vi "IronPythonSave.vi"(4 "Optical Spectrum":T1, 6 "Electrical Measurement":T6, 7 "Stress Motor Position":dbl, 8 "error in (no error)":errorcluster, 9 "Instrument Configuration":T3={"Instrument"=enum."Unknown Instrument", "Configuration"="Test Configuration"}, 10 "Workspace Info":T2={"Device Name"="test", "Device Info"="test", "Path"=path "C:/Users/gio/Desktop/test Python2Workspace/python2workspace_test.pmat"}, 11 "Function":T5) -> (0 "error out":errorcluster)   [LabVIEW 2014]
uses:
  Hardware Control/Parameter Analyzer/Electrical Data.ctl
  SaveData Function.ctl
  SaveData Instrument Configuration.ctl
  Instrument Sequence/Instrument List.ctl
  SaveData Workspace Info.ctl
  Hardware Control/Spectrometer/Spectral Data.ctl
  C:/IBM OEDUS/Measurements/Save Data/IronPythonSave/IronPythonSave.dll
  IronPythonSave/IronPythonSave.dll
panel:
  out "Activity Log":string
  out "concatenated string":string
  # "LICENSED MATERIALS – PROPERTY OF IBM\nCopyright IBM Corp. 2016,\nALL RIGHTS RESERVED"
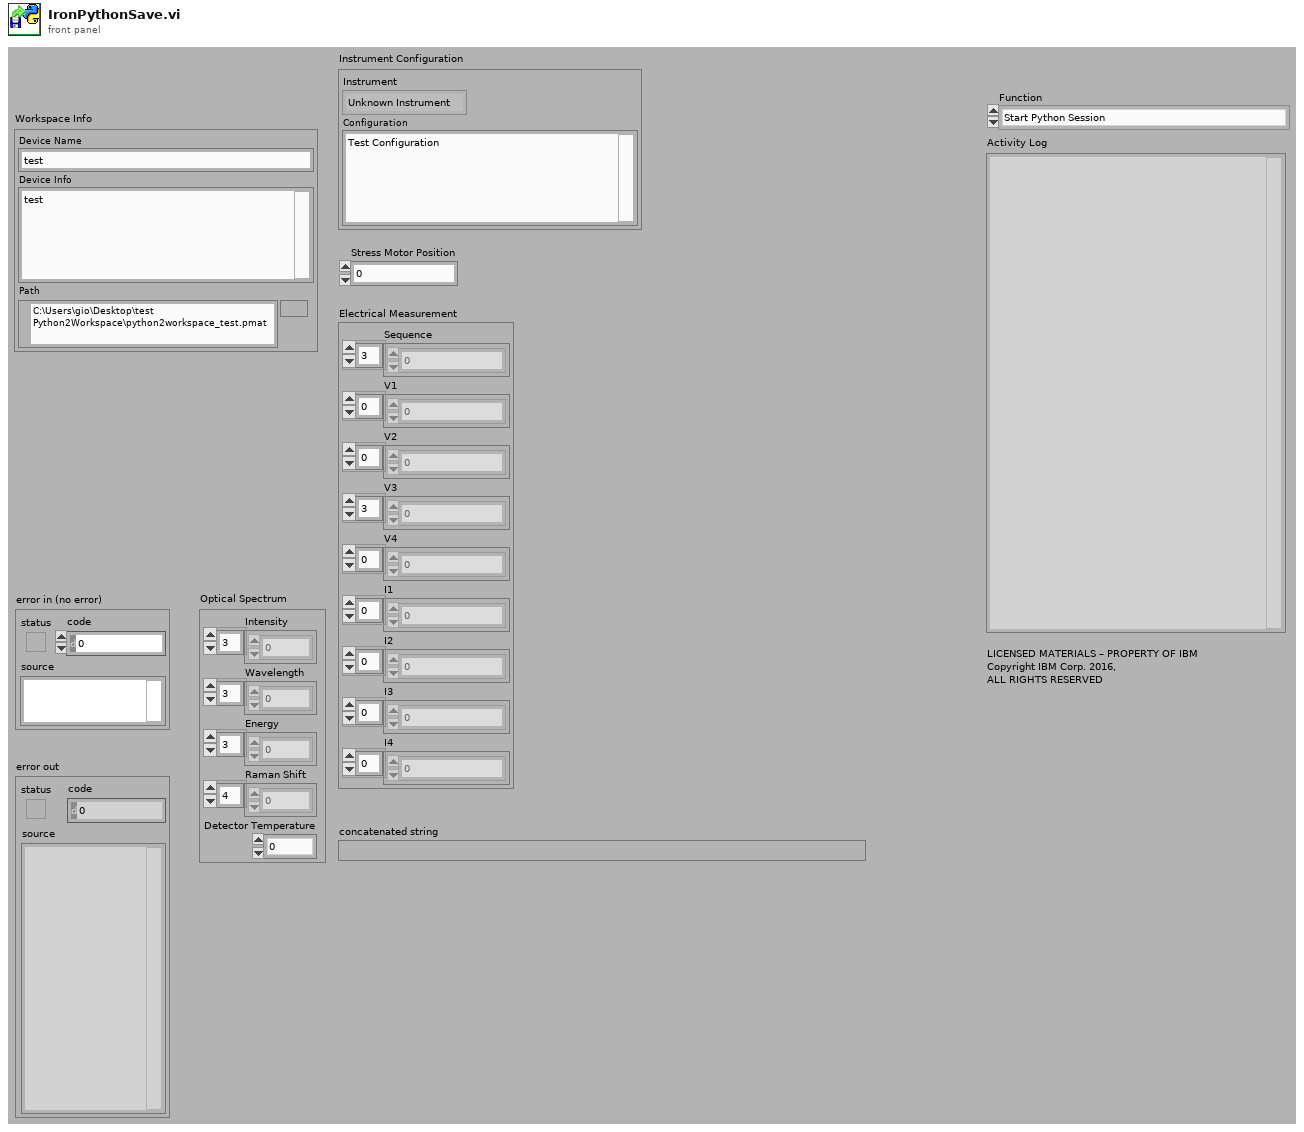
[diagram p1: front panel]
types:
  T1 = typedef "Spectral Data.ctl" = cluster{"Intensity":dbl[], "Wavelength":dbl[], "Energy":dbl[], "Raman Shift":dbl[], "Detector Temperature":dbl}
  T2 = typedef "SaveData Workspace Info.ctl" = cluster{"Device Name":string, "Device Info":string, "Path":path}
  T3 = typedef "SaveData Instrument Configuration.ctl" = cluster{"Instrument":T4, "Configuration":string}
  T4 = typedef "Instrument List.ctl" = enum32{"Unknown Instrument", "Switching Matrix", "Parameter Analyzer", "Optical Spectrometer", "Optoelectronic", "Autofocus"}
  T5 = typedef "SaveData Function.ctl" = enum16{"Start Python Session", "Set Data Structures to Default", "Append Stress Data", "Append Electrical Measurement", "Append Optical Spectrum", "Append Stress Measurement Step", "Append Instrument Sequence Step", "Set Instrument Configuration", "Set Stress Data", "Set Electrical Measurement", "Set Optical Spectum", "Save Electrical Measurement", "Save Optical Spectrum", "Save Optoelectronic Measurement", "Save Instrument Sequence", "Save Stress Measurement", "Pickle2Workspace", "Explore Variable Space", "Close"}
  T6 = typedef "Electrical Data.ctl" = cluster{"Sequence":dbl[], "V1":dbl[], "V2":dbl[], "V3":dbl[], "V4":dbl[], "I1":dbl[], "I2":dbl[], "I3":dbl[], "I4":dbl[]}
  T7 = enum32{"invalid app kind", "Development System", "Run Time System", "Student Edition", "Embedded LabVIEW", "Evaluation", "Custom"}
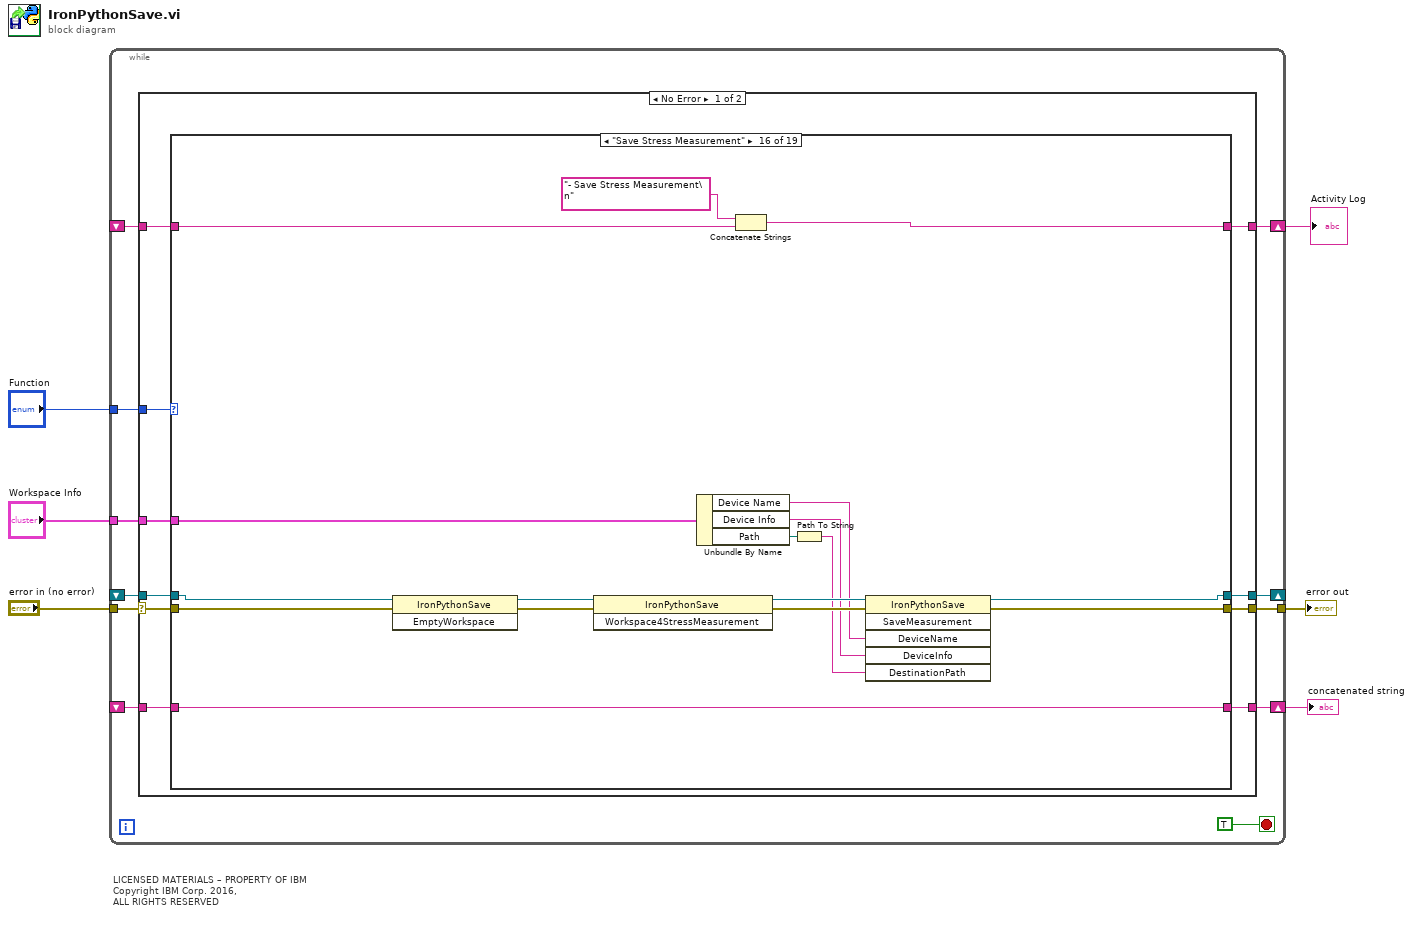
[diagram p0: block diagram]
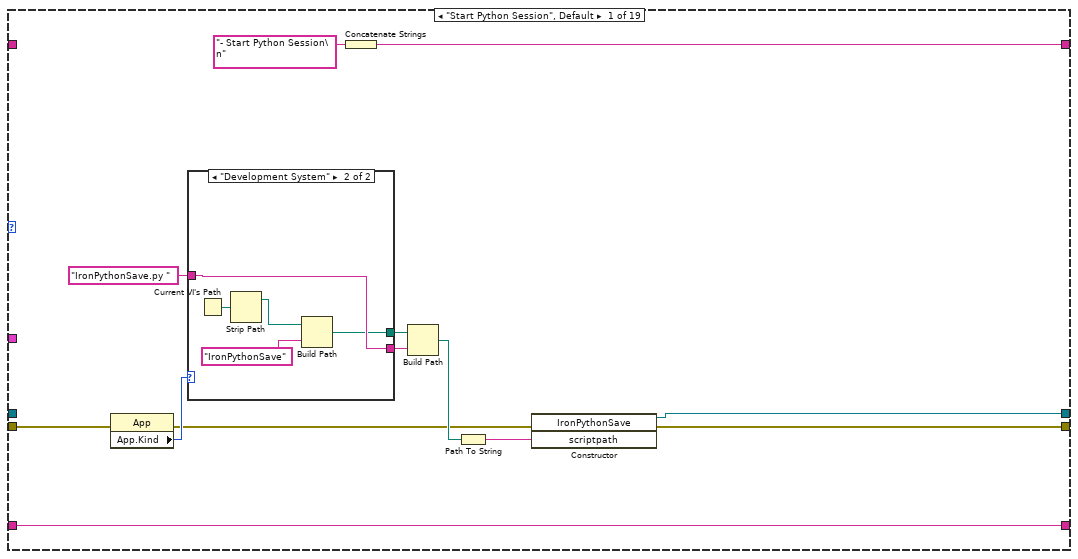
[diagram p2: hidden frame]
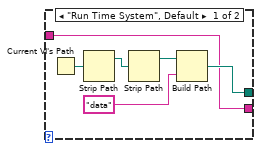
[diagram p3: hidden frame]
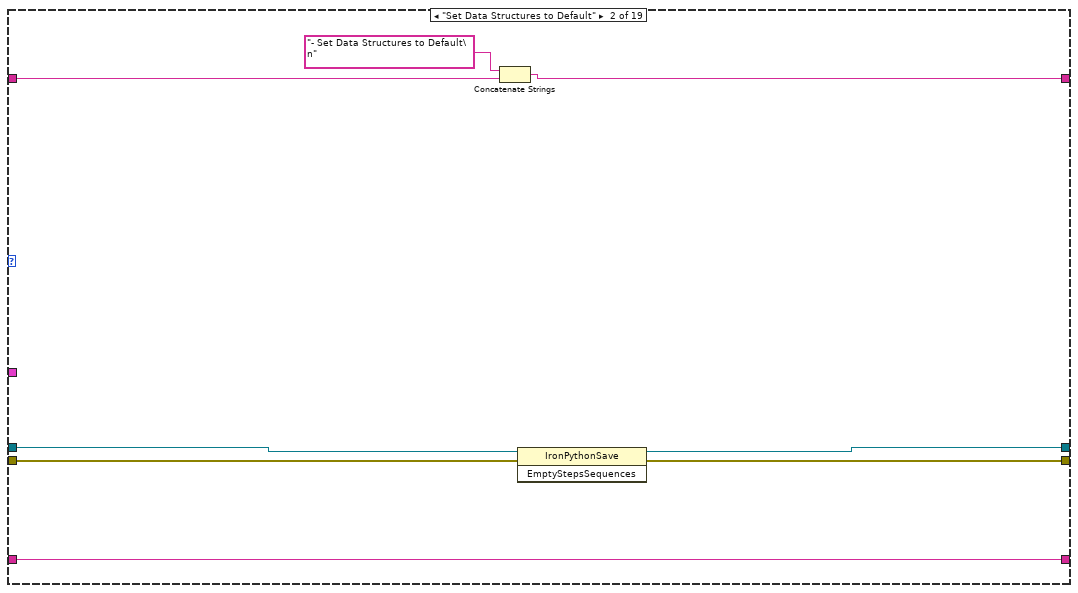
[diagram p4: hidden frame]
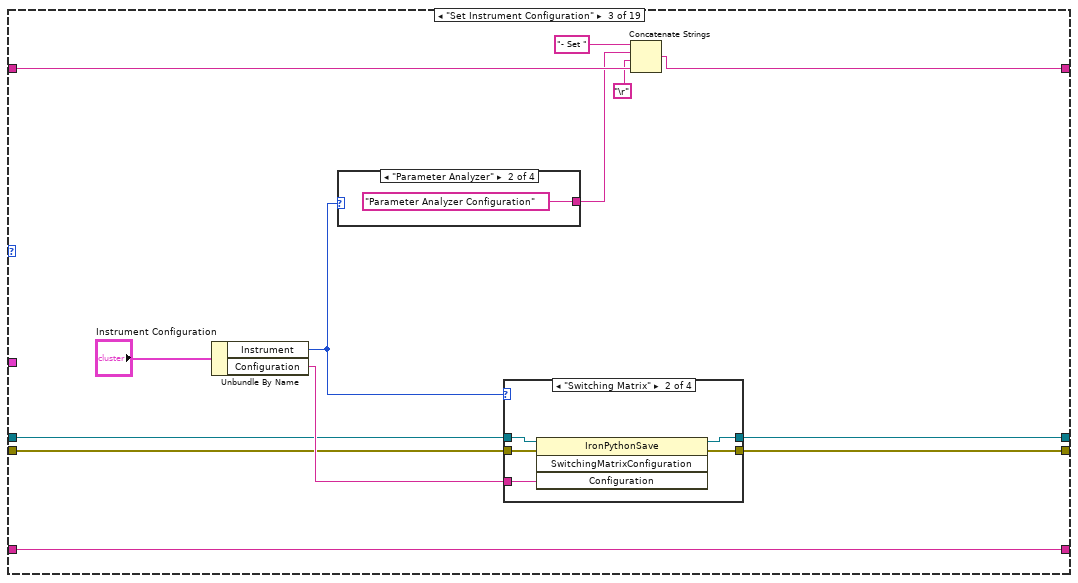
[diagram p5: hidden frame]
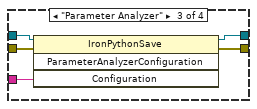
[diagram p7: hidden frame]
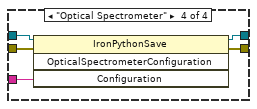
[diagram p8: hidden frame]
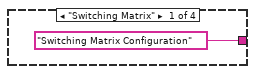
[diagram p9: hidden frame]
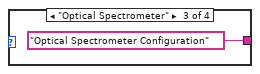
[diagram p10: hidden frame]
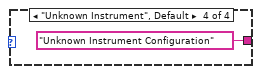
[diagram p11: hidden frame]
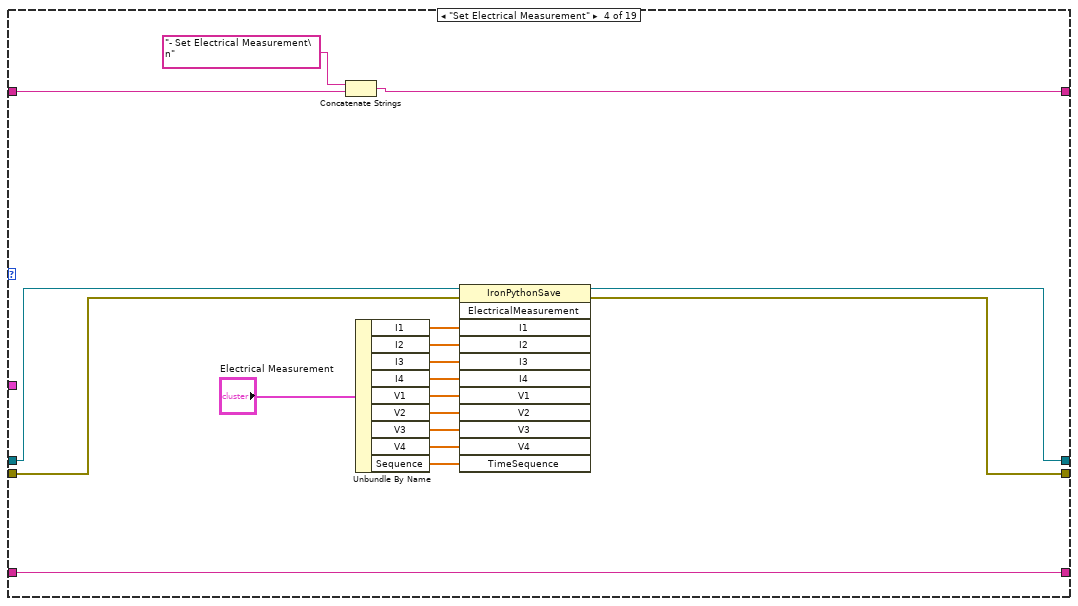
[diagram p12: hidden frame]
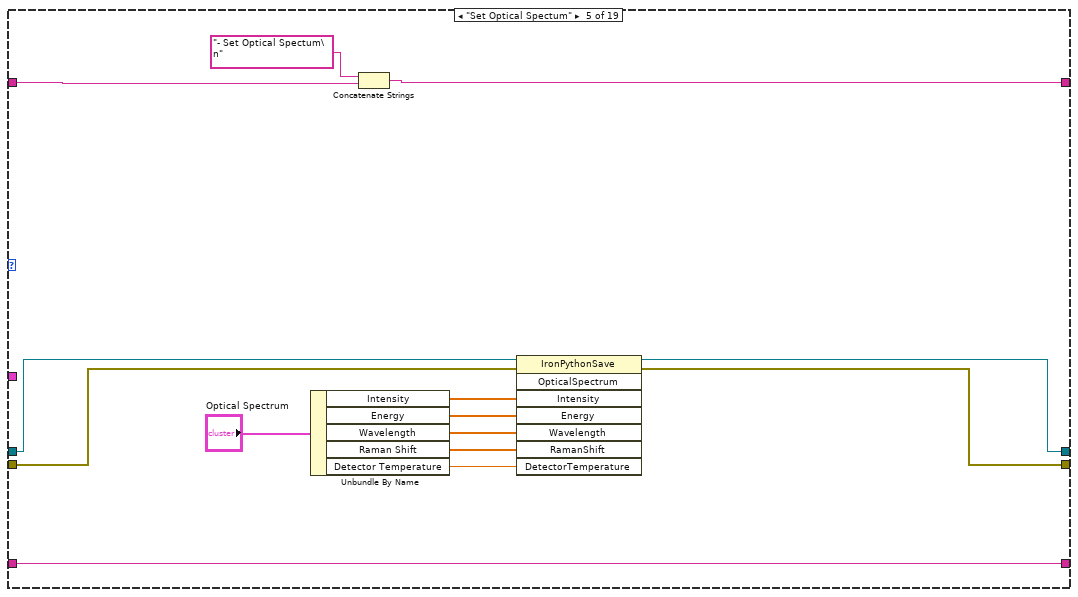
[diagram p13: hidden frame]
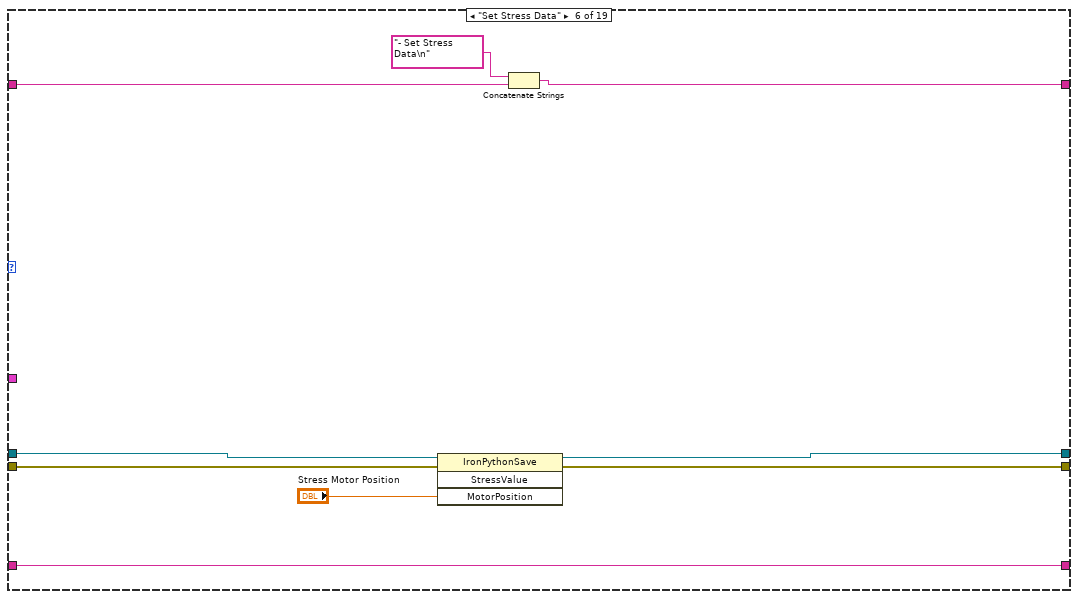
[diagram p14: hidden frame]
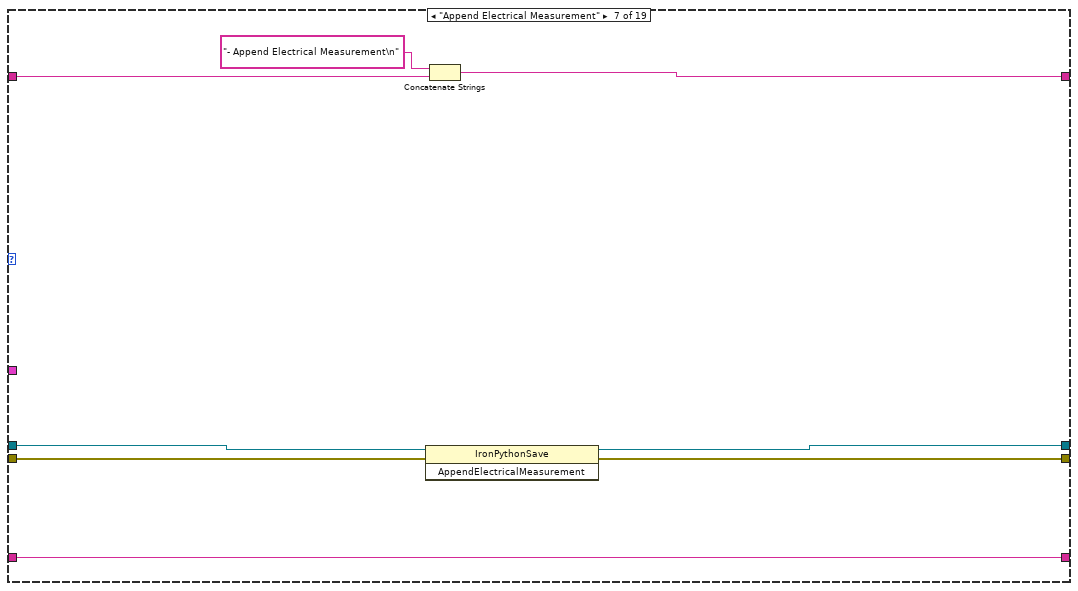
[diagram p15: hidden frame]
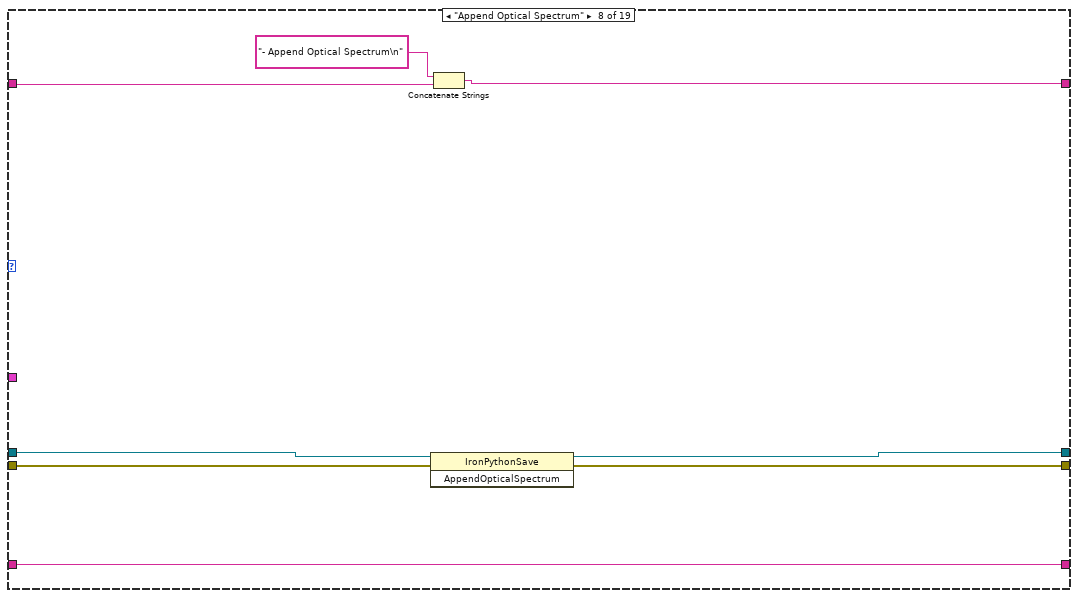
[diagram p16: hidden frame]
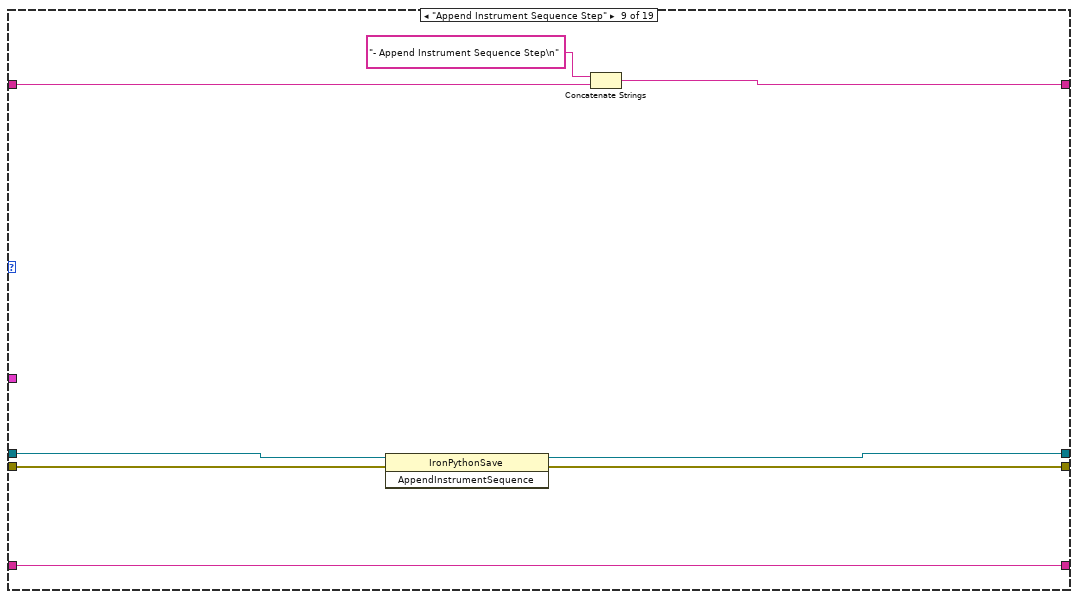
[diagram p17: hidden frame]
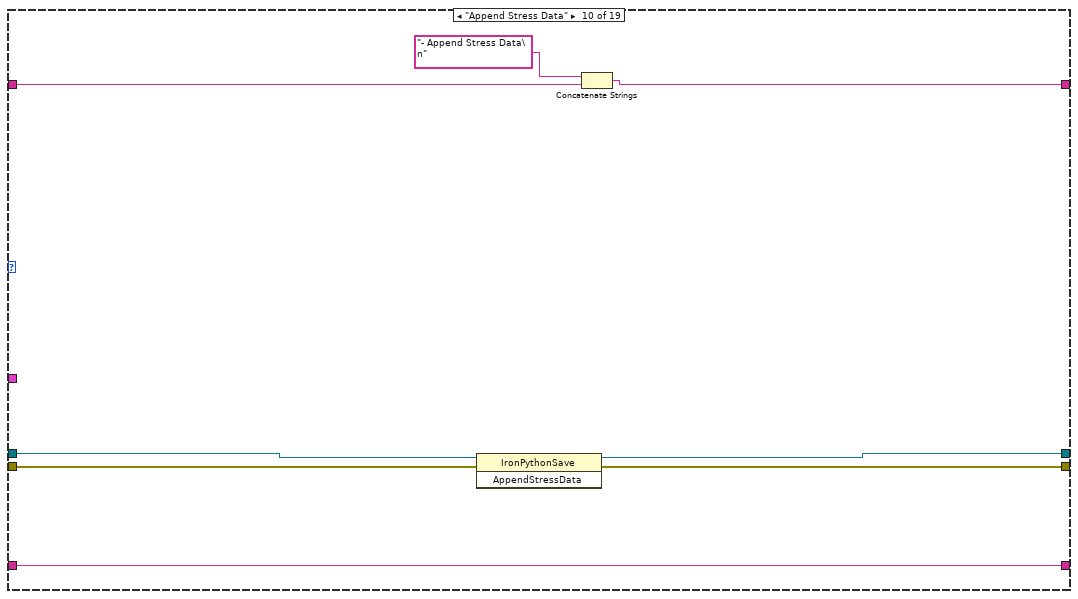
[diagram p18: hidden frame]
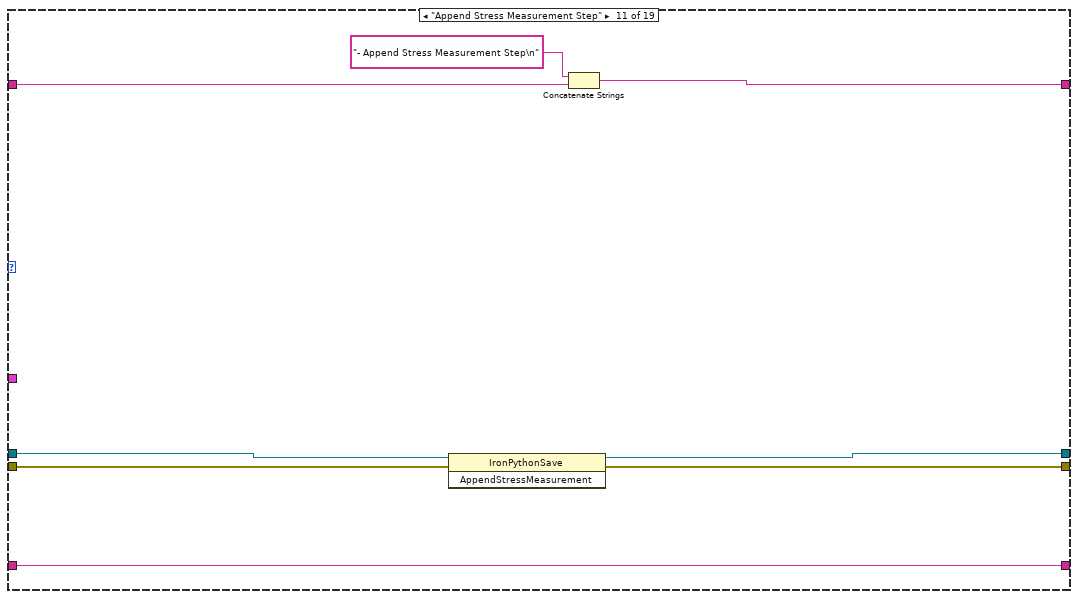
[diagram p19: hidden frame]
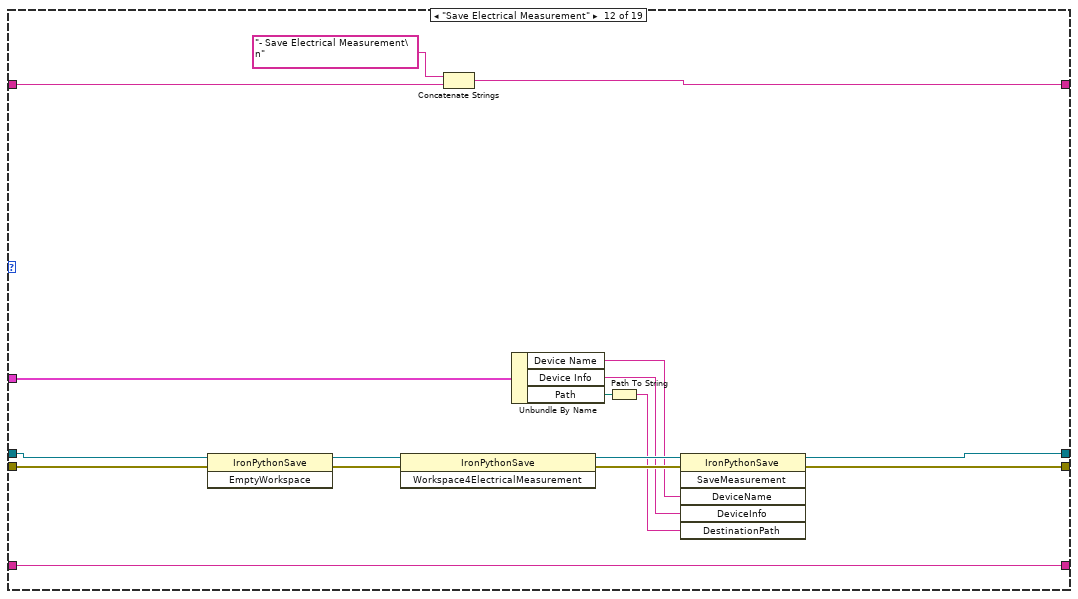
[diagram p20: hidden frame]
diagram:
  # "LICENSED MATERIALS – PROPERTY OF IBM\nCopyright IBM Corp. 2016,\nALL RIGHTS RESERVED"
  n1 = while {
    tunnel: "Workspace Info" -> [w17]
    tunnel: "Function" -> [w16]
    tunnel: [w15] -> w5
    tunnel: "error in (no error)" -> [w7]
    shift-right: [w13] -> _
    shift-left: _ -> [w12]
    shift-right: [w11] -> w2
    shift-left: _ -> [w10]
    shift-right: [w9] -> w1
    shift-left: _ -> [w8]
    stop <- TRUE stop-if-true
    n2 = case shown="No Error" w7 {
      selector: w7 -> [w24 w325]
      tunnel: w17 -> [w27 _]
      tunnel: w16 -> [w26 _]
      tunnel: [w25 w325] -> w15
      tunnel: [w23 w324] -> w13
      tunnel: w12 -> [w22 w324]
      tunnel: [w21 w323] -> w11
      tunnel: w10 -> [w20 w323]
      tunnel: w8 -> [w19 w322]
      tunnel: [w18 w322] -> w9
      frame No Error {
        n3 = case shown="\"Save Stress Measurement\"" w26 {
          tunnel: w27 -> [_ _ _ _ _ _ _ _ _ _ _ w190 w196 w217 w232 w247 _ _ w290]
          tunnel: w24 -> [w34 w54 w61 w105 w119 w129 w137 w145 w154 w161 w169 w184 w194 w216 w230 w249 w264 w269 w283]
          tunnel: [w28 w52 w64 w103 w117 w127 w136 w144 w151 w160 w167 w179 w192 w213 w229 w246 w263 w269 w288] -> w25
          tunnel: [w29 w53 w60 w104 w118 w126 w135 w143 w152 w159 w168 w178 w193 w214 w228 w245 w262 w270 w287] -> w23
          tunnel: w22 -> [_ w55 w62 w106 w120 w130 w138 w146 w153 w162 w170 w185 w195 w215 w231 w248 w262 w270 w287]
          tunnel: [w40 w59 w71 w110 w125 w134 w142 w150 w158 w166 w174 w189 w208 w227 w244 w261 w268 w272 w286] -> w21
          tunnel: w20 -> [w40 w59 w71 w110 w125 w134 w142 w150 w158 w166 w174 w189 w208 w227 w244 w261 w268 w272 _]
          tunnel: w19 -> [_ w58 w70 w109 w124 w132 w140 w148 w156 w165 w173 w188 w207 w226 w243 w260 w267 w271 w274]
          tunnel: [w39 w57 w69 w108 w123 w133 w141 w149 w157 w164 w172 w187 w206 w225 w242 w259 w266 w271 w275] -> w18
          frame "Start Python Session", Default {
            n4 = property class="App"(error in=w34) -> (error out=w31:errorcluster, "App.Kind"=w32:T7)  [unwired: 1 in, 1 out]
            n5 = case shown="\"Development System\"" w32 {
              tunnel: [w41 w50] -> w37
              tunnel: "IronPythonSave.py " ("command line") -> [w41 w50]
              tunnel: [w42 w48] -> w36
              frame "Run Time System", Default {
                n6 = Current VI's Path() -> (path=w46:path)
                n7 = Strip Path(path=w46) -> (stripped path=w45:path)  [unwired: 1 out]
                n8 = Strip Path(path=w45) -> (stripped path=w44:path)  [unwired: 1 out]
                n9 = Build Path(base path=w44, name or relative path="data" ("string")) -> (appended path=w42:path)
              }
              frame "Development System" {
                n10 = Current VI's Path() -> (path=w51:path)
                n11 = Strip Path(path=w51) -> (stripped path=w49:path)  [unwired: 1 out]
                n12 = Build Path(base path=w49, name or relative path="IronPythonSave") -> (appended path=w48:path)
              }
            }
            n13 = Concatenate Strings("- Start Python Session\n" ("string")) -> (w39:string)
            n14 = Build Path(base path=w36, name or relative path=w37) -> (appended path=w33:path)
            n15 = Path To String(path=w33) -> (string=w30:string)
            n16 = constructor class="IronPythonSave"(error in=w31, "scriptpath"=w30) -> (reference out=w29:refnum<k24>, error out=w28:errorcluster)  [unwired: 2 in, 2 out]
          }
          frame "Set Data Structures to Default" {
            n17 = Concatenate Strings("- Set Data Structures to Default\n" ("string"), w58) -> (w57:string)
            n18 = invoke class="IronPythonSave" method="EmptyStepsSequences"(reference=w55, error in=w54) -> (reference out=w53:refnum<k24>, error out=w52:errorcluster)  [unwired: 1 in, 1 out]
          }
          frame "Set Instrument Configuration" {
            n19 = Unbundle By Name("Instrument Configuration") -> ("Instrument"=w63:T4, "Configuration"=w65:string)
            n20 = case shown="\"Parameter Analyzer\"" w63 {
              tunnel: ["Switching Matrix Configuration" ("variable name") "Parameter Analyzer Configuration" ("variable name") "Optical Spectrometer Configuration" ("variable name") "Unknown Instrument Configuration" ("variable name")] -> w66
              frame "Switching Matrix" {
              }
              frame "Parameter Analyzer" {
              }
              frame "Optical Spectrometer" {
              }
              frame "Unknown Instrument", Default {
              }
            }
            n21 = case shown="\"Switching Matrix\"" w63 {
              tunnel: [w74 w76 w80 w86] -> w64
              tunnel: w65 -> [_ w75 w84 w85]
              tunnel: w62 -> [w73 w79 w82 w89]
              tunnel: w61 -> [w74 w78 w83 w88]
              tunnel: [w73 w77 w81 w87] -> w60
              frame "Unknown Instrument", Default {
              }
              frame "Switching Matrix" {
                n22 = invoke class="IronPythonSave" method="SwitchingMatrixConfiguration"(reference=w79, error in=w78, "Configuration"=w75) -> (reference out=w77:refnum<k24>, error out=w76:errorcluster)  [unwired: 1 in, 2 out]
              }
              frame "Parameter Analyzer" {
                n23 = invoke class="IronPythonSave" method="ParameterAnalyzerConfiguration"(reference=w82, error in=w83, "Configuration"=w84) -> (reference out=w81:refnum<k24>, error out=w80:errorcluster)  [unwired: 1 in, 2 out]
              }
              frame "Optical Spectrometer" {
                n24 = invoke class="IronPythonSave" method="OpticalSpectrometerConfiguration"(reference=w89, error in=w88, "Configuration"=w85) -> (reference out=w87:refnum<k24>, error out=w86:errorcluster)  [unwired: 1 in, 2 out]
              }
            }
            n25 = Concatenate Strings("- Set " ("string"), w66, "\r", w70) -> (w69:string)
          }
          frame "Set Electrical Measurement" {
            n26 = Concatenate Strings("- Set Electrical Measurement\n" ("string"), w109) -> (w108:string)
            n27 = Unbundle By Name("Electrical Measurement") -> ("I1"=w102:dbl[], "I2"=w101:dbl[], "I3"=w100:dbl[], "I4"=w99:dbl[], "V1"=w98:dbl[], "V2"=w97:dbl[], "V3"=w96:dbl[], "V4"=w95:dbl[], "Sequence"=w94:dbl[])
            n28 = invoke class="IronPythonSave" method="ElectricalMeasurement"(reference=w106, error in=w105, "I1"=w102, "I2"=w101, "I3"=w100, "I4"=w99, "V1"=w98, "V2"=w97, "V3"=w96, "V4"=w95, "TimeSequence"=w94) -> (reference out=w104:refnum<k24>, error out=w103:errorcluster)  [unwired: 1 in, 10 out]
          }
          frame "Set Optical Spectum" {
            n29 = Unbundle By Name("Optical Spectrum") -> ("Intensity"=w116:dbl[], "Energy"=w115:dbl[], "Wavelength"=w114:dbl[], "Raman Shift"=w113:dbl[], "Detector Temperature"=w112:dbl)
            n30 = Concatenate Strings("- Set Optical Spectum\n" ("string"), w124) -> (w123:string)
            n31 = invoke class="IronPythonSave" method="OpticalSpectrum"(reference=w120, error in=w119, "Intensity"=w116, "Energy"=w115, "Wavelength"=w114, "RamanShift"=w113, "DetectorTemperature"=w112) -> (reference out=w118:refnum<k24>, error out=w117:errorcluster)  [unwired: 1 in, 6 out]
          }
          frame "Set Stress Data" {
            n32 = invoke class="IronPythonSave" method="StressValue"(reference=w130, error in=w129, "MotorPosition"="Stress Motor Position") -> (reference out=w126:refnum<k24>, error out=w127:errorcluster)  [unwired: 1 in, 2 out]
            n33 = Concatenate Strings("- Set Stress Data\n" ("string"), w132) -> (w133:string)
          }
          frame "Append Electrical Measurement" {
            n34 = invoke class="IronPythonSave" method="AppendElectricalMeasurement"(reference=w138, error in=w137) -> (reference out=w135:refnum<k24>, error out=w136:errorcluster)  [unwired: 1 in, 1 out]
            n35 = Concatenate Strings("- Append Electrical Measurement\n" ("string"), w140) -> (w141:string)
          }
          frame "Append Optical Spectrum" {
            n36 = invoke class="IronPythonSave" method="AppendOpticalSpectrum"(reference=w146, error in=w145) -> (reference out=w143:refnum<k24>, error out=w144:errorcluster)  [unwired: 1 in, 1 out]
            n37 = Concatenate Strings("- Append Optical Spectrum\n" ("string"), w148) -> (w149:string)
          }
          frame "Append Instrument Sequence Step" {
            n38 = invoke class="IronPythonSave" method="AppendInstrumentSequence"(reference=w153, error in=w154) -> (reference out=w152:refnum<k24>, error out=w151:errorcluster)  [unwired: 1 in, 1 out]
            n39 = Concatenate Strings("- Append Instrument Sequence Step\n" ("string"), w156) -> (w157:string)
          }
          frame "Append Stress Data" {
            n40 = invoke class="IronPythonSave" method="AppendStressData"(reference=w162, error in=w161) -> (reference out=w159:refnum<k24>, error out=w160:errorcluster)  [unwired: 1 in, 1 out]
            n41 = Concatenate Strings("- Append Stress Data\n" ("string"), w165) -> (w164:string)
          }
          frame "Append Stress Measurement Step" {
            n42 = invoke class="IronPythonSave" method="AppendStressMeasurement"(reference=w170, error in=w169) -> (reference out=w168:refnum<k24>, error out=w167:errorcluster)  [unwired: 1 in, 1 out]
            n43 = Concatenate Strings("- Append Stress Measurement Step\n" ("string"), w173) -> (w172:string)
          }
          frame "Save Electrical Measurement" {
            n44 = invoke class="IronPythonSave" method="EmptyWorkspace"(reference=w185, error in=w184) -> (reference out=w183:refnum<k24>, error out=w182:errorcluster)  [unwired: 1 in, 1 out]
            n45 = invoke class="IronPythonSave" method="Workspace4ElectricalMeasurement"(reference=w183, error in=w182) -> (reference out=w181:refnum<k24>, error out=w180:errorcluster)  [unwired: 1 in, 1 out]
            n46 = Concatenate Strings("- Save Electrical Measurement\n" ("string"), w188) -> (w187:string)
            n47 = Unbundle By Name(w190) -> ("Device Name"=w177:string, "Device Info"=w176:string, "Path"=w191:path)
            n48 = Path To String(path=w191) -> (string=w175:string)
            n49 = invoke class="IronPythonSave" method="SaveMeasurement"(reference=w181, error in=w180, "DeviceName"=w177, "DeviceInfo"=w176, "DestinationPath"=w175) -> (reference out=w178:refnum<k24>, error out=w179:errorcluster)  [unwired: 1 in, 4 out]
          }
          frame "Save Optical Spectrum" {
            n50 = invoke class="IronPythonSave" method="EmptyWorkspace"(reference=w195, error in=w194) -> (reference out=w203:refnum<k24>, error out=w202:errorcluster)  [unwired: 1 in, 1 out]
            n51 = invoke class="IronPythonSave" method="Workspace4OpticalSPectrum"(reference=w203, error in=w202) -> (reference out=w201:refnum<k24>, error out=w200:errorcluster)  [unwired: 1 in, 1 out]
            n52 = Concatenate Strings("- Save Optical Spectrum\n" ("string"), w207) -> (w206:string)
            n53 = Unbundle By Name(w196) -> ("Device Name"=w199:string, "Device Info"=w198:string, "Path"=w204:path)
            n54 = Path To String(path=w204) -> (string=w197:string)
            n55 = invoke class="IronPythonSave" method="SaveMeasurement"(reference=w201, error in=w200, "DeviceName"=w199, "DeviceInfo"=w198, "DestinationPath"=w197) -> (reference out=w193:refnum<k24>, error out=w192:errorcluster)  [unwired: 1 in, 4 out]
          }
          frame "Save Optoelectronic Measurement" {
            n56 = invoke class="IronPythonSave" method="EmptyWorkspace"(reference=w215, error in=w216) -> (reference out=w209:refnum<k24>, error out=w210:errorcluster)  [unwired: 1 in, 1 out]
            n57 = invoke class="IronPythonSave" method="Workspace4ElectricalMeasurement"(reference=w209, error in=w210) -> (reference out=w212:refnum<k24>, error out=w211:errorcluster)  [unwired: 1 in, 1 out]
            n58 = Concatenate Strings("- Save Optoelectronic Measurement\n" ("string"), w226) -> (w225:string)
            n59 = invoke class="IronPythonSave" method="Workspace4OpticalSPectrum"(reference=w212, error in=w211) -> (reference out=w222:refnum<k24>, error out=w221:errorcluster)  [unwired: 1 in, 1 out]
            n60 = Unbundle By Name(w217) -> ("Device Name"=w220:string, "Device Info"=w219:string, "Path"=w223:path)
            n61 = Path To String(path=w223) -> (string=w218:string)
            n62 = invoke class="IronPythonSave" method="SaveMeasurement"(reference=w222, error in=w221, "DeviceName"=w220, "DeviceInfo"=w219, "DestinationPath"=w218) -> (reference out=w214:refnum<k24>, error out=w213:errorcluster)  [unwired: 1 in, 4 out]
          }
          frame "Save Instrument Sequence" {
            n63 = invoke class="IronPythonSave" method="EmptyWorkspace"(reference=w231, error in=w230) -> (reference out=w239:refnum<k24>, error out=w238:errorcluster)  [unwired: 1 in, 1 out]
            n64 = invoke class="IronPythonSave" method="Workspace4InstrumentSequence"(reference=w239, error in=w238) -> (reference out=w237:refnum<k24>, error out=w236:errorcluster)  [unwired: 1 in, 1 out]
            n65 = Unbundle By Name(w232) -> ("Device Name"=w235:string, "Device Info"=w234:string, "Path"=w240:path)
            n66 = Concatenate Strings("- Save Instrument Sequence\n" ("string"), w243) -> (w242:string)
            n67 = Path To String(path=w240) -> (string=w233:string)
            n68 = invoke class="IronPythonSave" method="SaveMeasurement"(reference=w237, error in=w236, "DeviceName"=w235, "DeviceInfo"=w234, "DestinationPath"=w233) -> (reference out=w228:refnum<k24>, error out=w229:errorcluster)  [unwired: 1 in, 4 out]
          }
          frame "Save Stress Measurement" {
            n69 = invoke class="IronPythonSave" method="EmptyWorkspace"(reference=w248, error in=w249) -> (reference out=w256:refnum<k24>, error out=w255:errorcluster)  [unwired: 1 in, 1 out]
            n70 = invoke class="IronPythonSave" method="Workspace4StressMeasurement"(reference=w256, error in=w255) -> (reference out=w254:refnum<k24>, error out=w253:errorcluster)  [unwired: 1 in, 1 out]
            n71 = Unbundle By Name(w247) -> ("Device Name"=w252:string, "Device Info"=w251:string, "Path"=w257:path)
            n72 = Concatenate Strings("- Save Stress Measurement\n" ("string"), w260) -> (w259:string)
            n73 = Path To String(path=w257) -> (string=w250:string)
            n74 = invoke class="IronPythonSave" method="SaveMeasurement"(reference=w254, error in=w253, "DeviceName"=w252, "DeviceInfo"=w251, "DestinationPath"=w250) -> (reference out=w245:refnum<k24>, error out=w246:errorcluster)  [unwired: 1 in, 4 out]
          }
          frame "Close" {
            n75 = Close Reference(reference=w262, error in (no error)=w264) -> (error out=w263:errorcluster)
            n76 = Concatenate Strings("- Python session Closed\n" ("string"), w267) -> (w266:string)
          }
          frame "Explore Variable Space" {
          }
          frame "Pickle2Workspace" {
            n77 = Unbundle By Name(w290) -> ("Path"=w289:path)
            n78 = property class="App"(error in=w283) -> (error out=w277:errorcluster, "App.Kind"=w278:T7)  [unwired: 1 in, 1 out]
            n79 = Path To String(path=w289) -> (string=w280:string)
            n80 = case shown="\"Development System\"" w278 {
              tunnel: [w300 w305] -> w286
              tunnel: [w298 w303] -> w285
              tunnel: w280 -> [w297 w304]
              tunnel: [w292 w302] -> w279
              tunnel: w277 -> [w291 w309]
              tunnel: [w291 w309] -> w276
              frame "Run Time System", Default {
                w298 = "Pickle2Workspace.py " ("command line")
                n81 = Current VI's Path() -> (path=w301:path)
                n82 = Strip Path(path=w301) -> (stripped path=w295:path)  [unwired: 1 out]
                n83 = Strip Path(path=w295) -> (stripped path=w294:path)  [unwired: 1 out]
                n84 = Build Path(base path=w294, name or relative path="data" ("string")) -> (appended path=w292:path)
                n85 = Concatenate Strings("python " ("command line"), w298, "" ("string"), w297) -> (w300:string)
              }
              frame "Development System" {
                w303 = "Pickle2Workspace.py " ("command line")
                n86 = Current VI's Path() -> (path=w308:path)
                n87 = Strip Path(path=w308) -> (stripped path=w302:path)  [unwired: 1 out]
                n88 = Concatenate Strings("python " ("command line"), w303, "" ("string"), w304) -> (w305:string)
              }
            }
            n89 = Concatenate Strings("- Pickle2Workspace\n" ("string"), w274) -> (w275:string)
            n90 = Build Path(base path=w279, name or relative path=w285) -> (appended path=w284:path)
            n91 = call <vilib>:"Check if File or Folder Exists.vi"("error in (no error)"=w276, "path"=w284) -> ("error out"=w282:errorcluster, "file or folder exists?"=w281:bool)  [unwired: 7 in, 1 out]
            n92 = case shown="True" w281 {
              tunnel: w282 -> [w313 w321]
              tunnel: [w312 w320] -> w288
              tunnel: w279 -> [w311 w319]
              tunnel: w286 -> [w310 w318]
              frame False {
                n93 = Path To String(path=w311) -> (string=w315:string)
                n94 = Concatenate Strings(w315, "   \\   " ("string"), w310) -> (w316:string)
                n95 = call "Dialog.vi"("error in (no error)"=w313, "message"=w316) -> ("error out"=w312:errorcluster)  [unwired: 9 in]
              }
              frame True {
                n96 = call <vilib>:"System Exec.vi"("run minimized? (F)"=TRUE, "error in (no error)"=w321, "working directory"=w319, "command line"=w318) -> ("error out"=w320:errorcluster)  [unwired: 2 in, 5 out]
              }
            }
          }
        }
      }
      frame Error {
      }
    }
  }
  "error out" <- w5
  "concatenated string" <- w2
  "Activity Log" <- w1
